vi "Python_Close.vi"(2 "error in (no error)":errorcluster) -> (0 "error out":errorcluster)   [LabVIEW 2025]
panel:
  out "Paths Erased":path[](array[path])
  out "Array":errorcluster[](array[cluster])
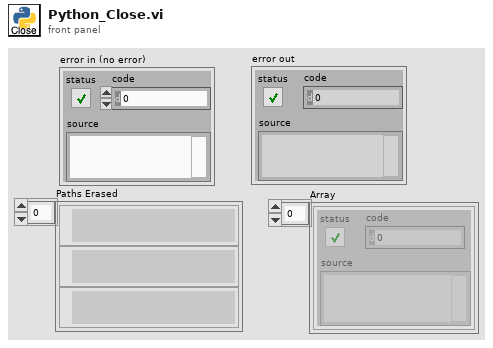
[diagram p1: front panel]
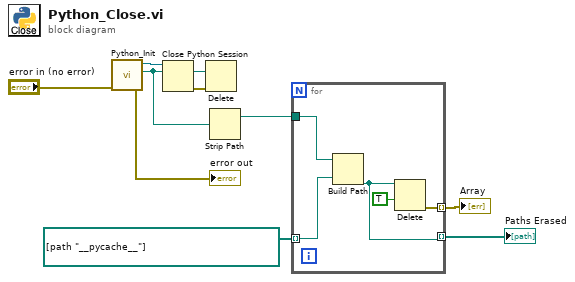
[diagram p0: block diagram]
diagram:
  n1 = call "Python_Init.vi"("error in (no error)"="error in (no error)") -> ("Refnum out"=w9:refnum<k35>, "code"=w6:path, "error out"=→"error out":errorcluster)  [unwired: 3 in]
  n2 = Close Python Session(session in=w9) -> (11:w8:errorcluster)  [unwired: 1 in]
  n3 = Delete(path (use dialog)=w6, error in=w8) -> ()  [unwired: 3 in, 3 out]
  n4 = Strip Path(path=w6) -> (stripped path=w1:path)  [unwired: 1 out]
  n5 = for {
    tunnel: path[] [path "__pycache__"] -> [w11] mode=indexing
    tunnel: w1 -> [w13]
    tunnel: [w12] -> w3 mode=indexing
    tunnel: [w10] -> w2 mode=indexing
    n6 = Build Path(base path=w13, name or relative path=w11) -> (appended path=w10:path)
    n7 = Delete(path (use dialog)=w10, entire hierarchy (F)=TRUE ("confirm (F)")) -> (error out=w12:errorcluster)  [unwired: 3 in, 2 out]
  }
  "Array" <- w3
  "Paths Erased" <- w2
